vi "List Dependencies.vi"(8 "error in (no error)":errorcluster, 11 "Attribute.Dependencies in":refnum<class "Attribute.Dependencies.lvclass">) -> (0 "error out":errorcluster, 2 "Dependencies":T1[](array[typedef]), 3 "Attribute.Dependencies out":refnum<class "Attribute.Dependencies.lvclass">)   [LabVIEW 2021, in "smo.lvlib" / "Attribute.Dependencies.lvclass"]
uses:
  Attribute.Dependencies.lvclass
  DependencyAttr--Cluster.ctl
  SMO/SMO.lvclass
  Attribute.Dependencies.lvclass/Attribute.Dependencies.ctl
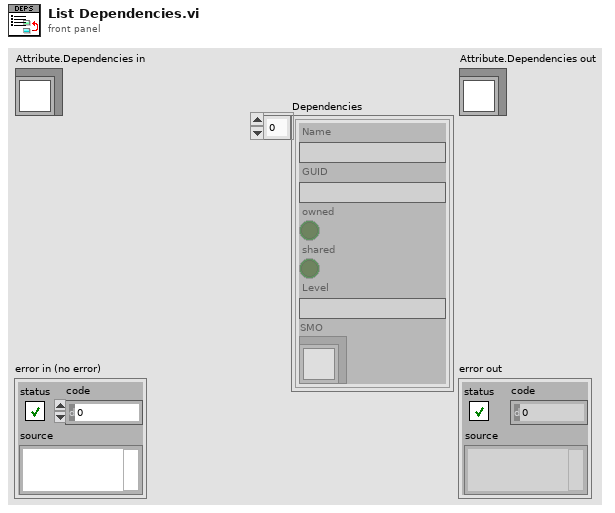
[diagram p1: front panel]
types:
  T1 = typedef "smo.lvlib/Attribute.Dependencies.lvclass/DependencyAttr--Cluster.ctl" = cluster{"Name":string, "GUID":string, "owned":bool, "shared":bool, "Level":string, "SMO":refnum<class "SMO.lvclass">}
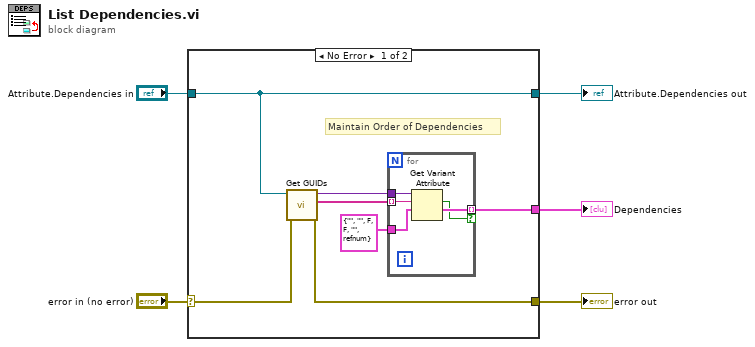
[diagram p0: block diagram]
diagram:
  n1 = case shown="No Error" "error in (no error)" {
    selector: "error in (no error)" -> [w8 w19]
    tunnel: [w7 w19] -> w4
    tunnel: [w6 w18] -> w2
    tunnel: "Attribute.Dependencies in" -> [w6 w18]
    tunnel: [w12 _] -> w1
    frame No Error {
      # "Maintain Order of Dependencies"
      n2 = call "Get GUIDs.vi"("error in (no error)"=w8, "Attribute.Dependencies"=w6) -> ("error out"=w7:errorcluster, "GUIDs"=w10:string[], "Variant"=w11:variant)  [unwired: 7 in]
      n3 = for {
        tunnel: T1 {"Name"="", "GUID"="", "owned"=FALSE, "shared"=FALSE, "Level"="", "SMO"=refnum} ("Dependency") -> [w15]
        tunnel: [w14] -> w12 mode=indexing if=w13
        tunnel: w11 -> [w17]
        tunnel: w10 -> [w16] mode=indexing
        n4 = Get Variant Attribute(Variant=w17, name=w16, default value (empty Variant)=w15) -> (found=w13:bool, value=w14:T1)  [unwired: 1 in, 2 out]
      }
    }
    frame Error {
    }
  }
  "error out" <- w4
  "Attribute.Dependencies out" <- w2
  "Dependencies" <- w1
